vi "Trajectory Variables.vi"() -> ()   [LabVIEW 2020]
panel:
  in  "Traj State":u16(ring)
  out "Gyro Cont":dbl format="%_6g"
  in  "TrajectoryFiles":string[](array[string])
  out "Traj_Total_Time":dbl format="%_6g"
  out "Traj_Total_States":dbl format="%_6g"
  out "VelocityRightTarget":dbl format="%_6g"
  out "VelocityLeftTarget":dbl format="%_6g"
  out "DistanceLeft":dbl format="%_6g"
  out "VelocityLeft":dbl format="%_6g"
  out "DistanceRight":dbl format="%_6g"
  out "VelocityRight":dbl format="%_6g"
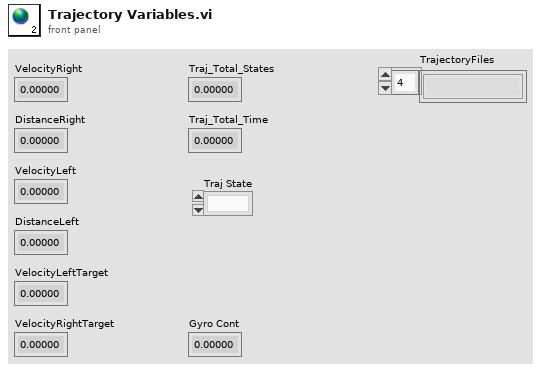
[diagram p1: front panel]
diagram:
